vi "Convert Images.vi"(0 "Image In":T1, 5 "Max Value":dbl=15.0 format="%#_13g", 7 "Min Value":dbl, 11 "Error in (no error)":errorcluster) -> (4 "Image Out":T1, 15 "Error out":errorcluster)   [LabVIEW 2022 SP3]
uses:
  <vilib>/vision/Image Controls.llb/IMAQ Image.ctl
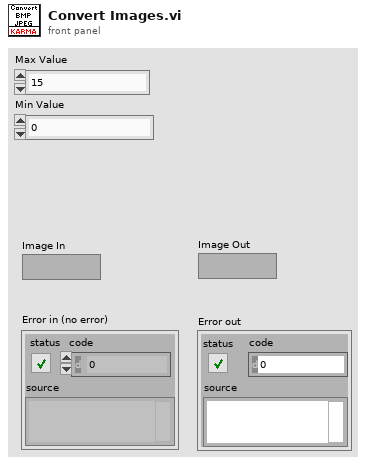
[diagram p1: front panel]
types:
  T1 = typedef "IMAQ Image.ctl" = refnum<image>
  T2 = typedef "Image Type" = u32
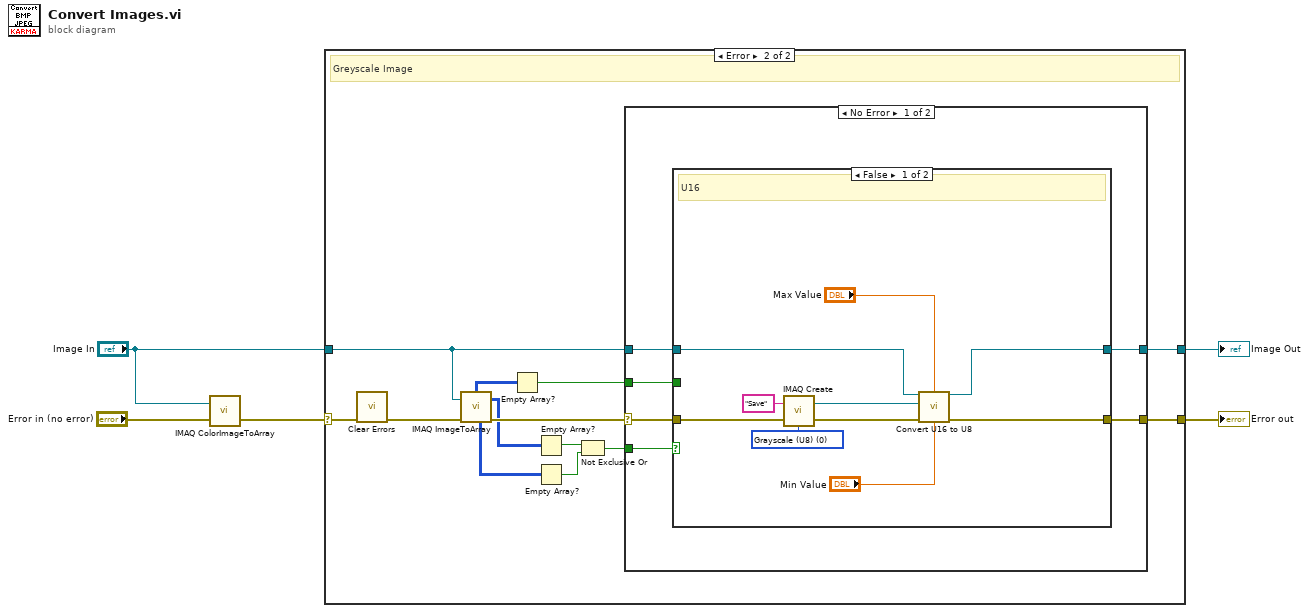
[diagram p0: block diagram]
diagram:
  n1 = call "IMAQ ColorImageToArray"("Image"="Image In", "error in (no error)"="Error in (no error)") -> ("error out"=w3:errorcluster)  [unwired: 2 in, 2 out]
  n2 = case shown="Error" w3 {
    selector: w3 -> [w6 w18]
    tunnel: "Image In" -> [w7 w15]
    tunnel: [w7 w14] -> w2
    tunnel: [w6 w16] -> w1
    frame No Error {
      # "Color Image"
    }
    frame Error {
      # "Greyscale Image"
      n3 = call <vilib>:"Clear Errors.vi"("error in (no error)"=w18) -> ("error out"=w13:errorcluster)  [unwired: 5 in, 1 out]
      n4 = call "IMAQ ImageToArray"("error in (no error)"=w13, "Image"=w15) -> ("Image Pixels (U16)"=w19:u16[][], "error out"=w17:errorcluster, "Image Pixels (U8)"=w20:u8[][], "Image Pixels (I16)"=w12:i16[][])  [unwired: 2 in, 1 out]
      n5 = Empty Array?(array=w20) -> (empty?=w11:bool)
      n6 = Empty Array?(array=w12) -> (empty?=w10:bool)
      n7 = Empty Array?(array=w19) -> (empty?=w9:bool)
      n8 = Not Exclusive Or(1:w9, 2:w10) -> (0:w8:bool)
      n9 = case shown="No Error" w17 {
        selector: w17 -> [w24 w46]
        tunnel: w8 -> [w26 _]
        tunnel: w11 -> [w25 _]
        tunnel: [w23 w46] -> w16
        tunnel: w15 -> [w22 w47]
        tunnel: [w21 w47] -> w14
        frame No Error {
          n10 = case shown="False" w26 {
            tunnel: w25 -> [_ w41]
            tunnel: w24 -> [w34 w40]
            tunnel: [w30 w39] -> w23
            tunnel: w22 -> [w33 w38]
            tunnel: [w29 w37] -> w21
            frame False {
              w35 = T2 0 items=["Grayscale (U8)", "Grayscale (I16)", "Grayscale (SGL)", "Complex (CSG)", "RGB (U32)", "HSL (U32)", "RGB (U64)", "Grayscale (U16)"] ("Image Type")
              # "U16"
              n11 = call "IMAQ Create"("Image Name"="Save", "Image Type"=w35, "error in (no error)"=w34) -> ("New Image"=w32:T1, "error out"=w31:errorcluster)  [unwired: 2 in]
              n12 = call "Convert U16 to U8.vi"("Image Src"=w33, "Max Value"="Max Value", "Image Dst"=w32, "Error in (no error)"=w31, "Min Value"="Min Value") -> ("Image Out"=w29:T1, "Error out"=w30:errorcluster)  [unwired: 8 in, 1 out]
            }
            frame True {
              # "Not U16"
              n13 = case shown="True" w41 {
                tunnel: w40 -> [w43 w45]
                tunnel: [w43 w45] -> w39
                tunnel: w38 -> [w42 w44]
                tunnel: [w42 w44] -> w37
                frame False {
                  # "U8"
                }
                frame True {
                  # "Unknown Image Type"
                }
              }
            }
          }
        }
        frame Error {
        }
      }
    }
  }
  "Image Out" <- w2
  "Error out" <- w1
